vi "Write ulDGNr.vi"(8 "error in (no error)":errorcluster, 9 "ulSlotNr":i32, 10 "ulDGNr":i32, 11 "BME_DG_Base in":refnum<class "BME_DG_Base.lvclass">) -> (0 "error out":errorcluster, 3 "BME_DG_Base out":refnum<class "BME_DG_Base.lvclass">)   [LabVIEW 2009, in "BME_DG_Base.lvclass"]
uses:
  BME_DG_Base.lvclass
  BME_DG_Base.lvclass/BME_DG_Base.ctl
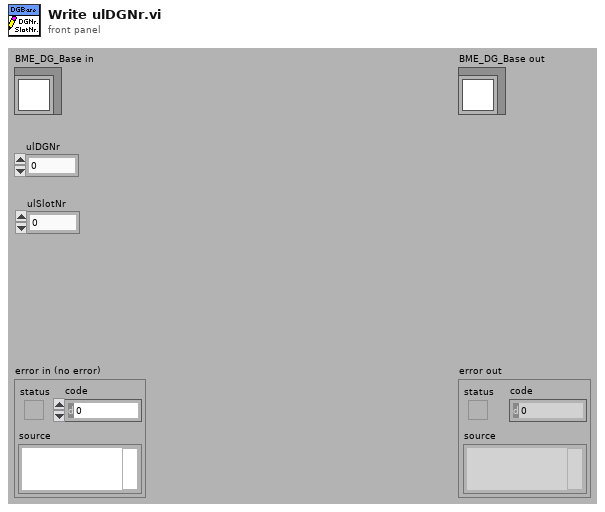
[diagram p1: front panel]
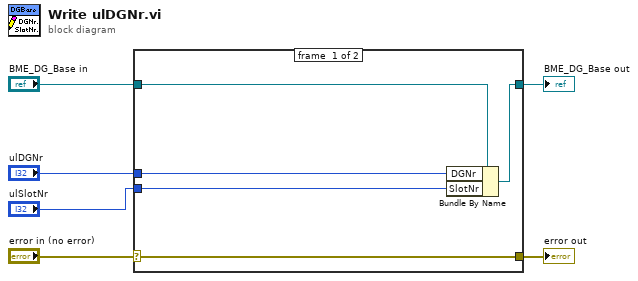
[diagram p0: block diagram]
diagram:
  n1 = case shown="No Error" "error in (no error)" {
    selector: "error in (no error)" -> [w11 w12]
    tunnel: [w11 w12] -> w5
    tunnel: [w9 w13] -> w3
    tunnel: "BME_DG_Base in" -> [w10 w13]
    tunnel: "ulDGNr" -> [w8 _]
    tunnel: "ulSlotNr" -> [w7 _]
    frame #0 {
      n2 = Bundle By Name(cluster=w10, "DGNr"=w8, "SlotNr"=w7) -> (w9:refnum<class "BME_DG_Base.lvclass">)
    }
    frame #1 {
    }
  }
  "error out" <- w5
  "BME_DG_Base out" <- w3
